vi "EnableSecondaryPorts.vi"(8 "error in (no error)":errorcluster, 10 "Session in":refnum<k21>="localhost", 11 "Network Configuration":T1[](array[typedef]) {"IP Address Request Mode" items=["Static"=1, "DHCP/Link Local"=2, "Link-Local Only"=4, "DHCP Only"=8]; "Adapter Mode" items=["Disabled"=1, "TCP/IP Ethernet"=2, "Deterministic"=4, "EtherCAT"=8, "TCP/IP WLAN Connect"=32, "TCP/IP WLAN Create"=64]}) -> (0 "error out":errorcluster, 2 "reboot required":bool)   [LabVIEW 2017]
uses:
  <vilib>/nisyscfg/nisyscfg.lvlib
  <resource>/objmgr/niflexriosae.rc
  <resource>/objmgr/nicriosae.rc
  <vilib>/nisyscfg/Find Hardware.vi
  <vilib>/nisyscfg/Close (Filter).vi
  <vilib>/nisyscfg/Close (System).vi
  <vilib>/nisyscfg/Close (Hardware).vi
  <vilib>/nisyscfg/Save Changes (Hardware).vi
  <vilib>/addons/InsightCM/Utilities/Networking/controls/NetworkCfg.ctl
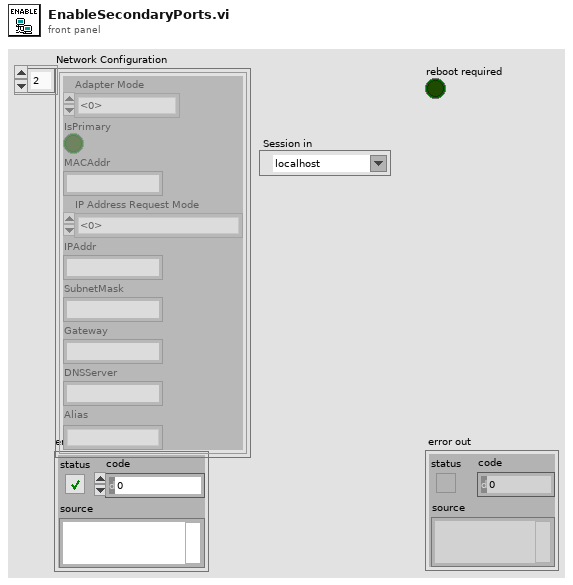
[diagram p1: front panel]
types:
  T1 = typedef "NetworkCfg.ctl" = cluster{"Adapter Mode":u32, "IsPrimary":bool, "MACAddr":string, "IP Address Request Mode":u32, "IPAddr":string, "SubnetMask":string, "Gateway":string, "DNSServer":string, "Alias":string}
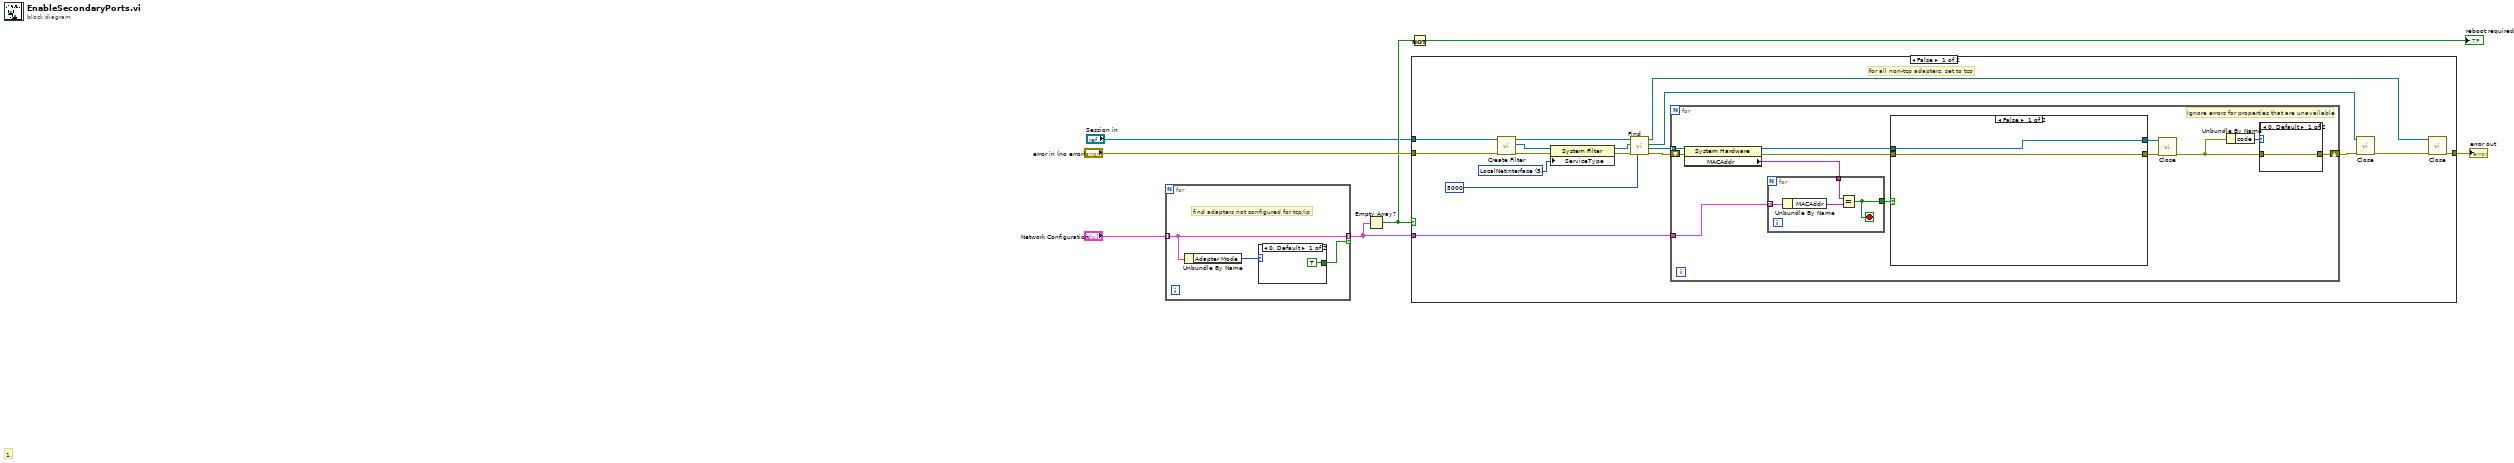
[diagram p0: block diagram]
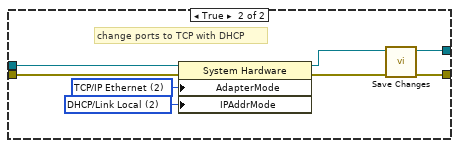
[diagram p2: hidden frame]
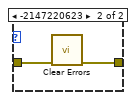
[diagram p3: hidden frame]
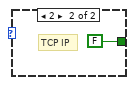
[diagram p5: hidden frame]
diagram:
  # "1."
  n1 = for {
    tunnel: "Network Configuration" -> [w9] mode=indexing
    tunnel: [w9] -> w4 mode=indexing if=w8
    # "find adapters not configured for tcp/ip"
    n2 = Unbundle By Name(w9) -> ("Adapter Mode"=w10:u32)
    n3 = case shown="0, Default" w10 {
      tunnel: [TRUE FALSE] -> w8
      frame 0, Default {
      }
      frame 2 {
        # "TCP IP"
      }
    }
  }
  n4 = Empty Array?(array=w4) -> (empty?=w3:bool)
  n5 = Not(x=w3) -> (.not. x?=→"reboot required":bool)
  n6 = case shown="False" w3 {
    tunnel: "error in (no error)" -> [w14 w59]
    tunnel: [w18 w59] -> w6
    tunnel: w4 -> [w17 _]
    tunnel: "Session in" -> [w13 _]
    frame False {
      w28 = u32 5 items=["mDnsNiTcp", "mDnsNiRealtime", "mDnsNiSysapi", "mDnsNiHttp", "LocalSystem", "LocalNetInterface", "LocalTimeKeeper", "LocalTimeSource", "mDnsLxi"] ("Service Type")
      # "for all non-tcp adapters, set to tcp"
      n7 = call <vilib>:"Create Filter.vi"("error in (no error)"=w14, "Session in"=w13) -> ("error out"=w27:errorcluster, "Filter out"=w29:refnum<k20>, "Session out"=w25:refnum<k21>)  [unwired: 7 in]
      n8 = property class="System Filter"(reference=w29, error in=w27, "ServiceType"=w28) -> (reference out=w24:refnum<k20>, error out=w26:errorcluster)
      n9 = call-poly <vilib>:"Find.vi"("Remote Timeout (300,000 ms)"=u32 5000 ("Timeout (milliseconds)"), "error in (no error)"=w26, "Filter in"=w24, "Session in"=w25) -> ("error out"=w22:errorcluster, "Resources out"=w23:refnum<k20>[], "Filter out"=w20:refnum<k20>, "Session out"=w16:refnum<k21>)  [unwired: 4 in]
      n10 = for {
        tunnel: w23 -> [w40] mode=indexing
        shift-right: [w37] -> w21
        shift-left: w22 -> [w41]
        tunnel: w17 -> [w36]
        # "Ignore errors for properties that are unavailable"
        n11 = property class="System Hardware"(reference=w40, error in=w41) -> (reference out=w33:refnum<k20>, error out=w32:errorcluster, "MACAddr"=w35:string)
        n12 = for {
          tunnel: w36 -> [w45] mode=indexing
          tunnel: w35 -> [w44]
          tunnel: [w42] -> w34
          stop <- w42 stop-if-true
          n13 = Unbundle By Name(w45) -> ("MACAddr"=w43:string)
          n14 = Equal?(x=w44, y=w43) -> (x = y?=w42:bool)
        }
        n15 = case shown="False" w34 {
          tunnel: w33 -> [w47 w55]
          tunnel: w32 -> [w46 w54]
          tunnel: [w47 w49] -> w31
          tunnel: [w46 w48] -> w30
          frame False {
          }
          frame True {
            w52 = u32 2 items=["Static"=1, "DHCP/Link Local"=2, "Link-Local Only"=4, "DHCP Only"=8] ("Network Adapters:TCP/IP:IP Address Request Mode")
            w53 = u32 2 items=["Disabled"=1, "TCP/IP Ethernet"=2, "Deterministic"=4, "EtherCAT"=8, "TCP/IP WLAN Connect"=32, "TCP/IP WLAN Create"=64] ("Network Adapters:Adapter Mode")
            # "change ports to TCP with DHCP"
            n16 = property class="System Hardware"(reference=w55, error in=w54, "AdapterMode"=w53, "IPAddrMode"=w52) -> (reference out=w50:refnum<k20>, error out=w51:errorcluster)
            n17 = call-poly <vilib>:"Save Changes.vi"("error in (no error)"=w51, "Resource in"=w50) -> ("error out"=w48:errorcluster, "Resource out"=w49:refnum<k20>)  [unwired: 6 in, 2 out]
          }
        }
        n18 = call-poly <vilib>:"Close.vi"("error in (no error)"=w30, "Resource in"=w31) -> ("error out"=w38:errorcluster)  [unwired: 9 in]
        n19 = Unbundle By Name(w38) -> ("code"=w39:i32)
        n20 = case shown="0, Default" w39 {
          tunnel: [w56 w58] -> w37
          tunnel: w38 -> [w56 w57]
          frame 0, Default {
          }
          frame -2147220623 {
            n21 = call <vilib>:"Clear Errors.vi"("error in (no error)"=w57) -> ("error out"=w58:errorcluster)  [unwired: 5 in, 1 out]
          }
        }
      }
      n22 = call-poly <vilib>:"Close.vi"("error in (no error)"=w21, "Filter in"=w20) -> ("error out"=w15:errorcluster)  [unwired: 9 in]
      n23 = call-poly <vilib>:"Close.vi"("error in (no error)"=w15, "Session in"=w16) -> ("error out"=w18:errorcluster)  [unwired: 9 in]
    }
    frame True {
    }
  }
  "error out" <- w6
